vi "Set Certificate Status.vi"(8 "error in (no error)":errorcluster, 9 "Certificate Status":T1, 10 "Certificate ID":string, 11 "IoT Session in":refnum<class "IoT Session.lvclass">) -> (0 "error out":errorcluster, 3 "IoT Session out":refnum<class "IoT Session.lvclass">)   [LabVIEW 2015, in "NI_AWS_IoT.lvlib" / "IoT Session.lvclass"]
uses:
  IoT Session.lvclass
  Certificate Status.ctl
  Core/HTTP Request/Request Options.ctl
  Core/HTTP Request/Name Value Pair.ctl
  Core/HTTP Request/Region handling.ctl
  Core/HTTP Request/URL formatting.ctl
  Core/HTTP Request/HTTP Request.lvclass
  NI_AWS_IoT.lvlib
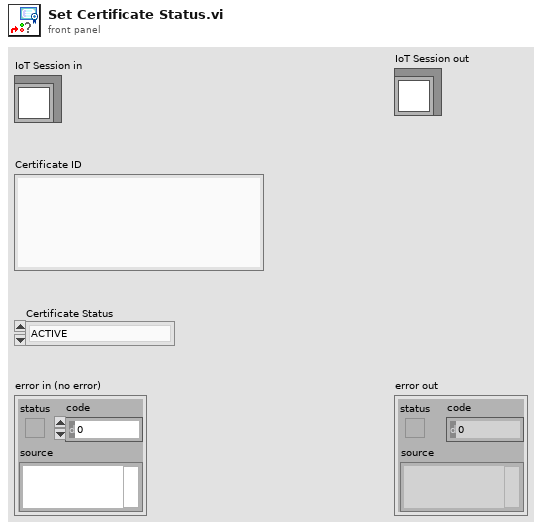
[diagram p1: front panel]
types:
  T1 = typedef "NI_AWS_IoT.lvlib/Certificate Status.ctl" = enum16{"ACTIVE", "INACTIVE", "REVOKED", "PENDING_TRANSFER", "REGISTER_INACTIVE", "PENDING_ACTIVATION"}
  T2 = typedef "NI_AWS_Core.lvlib/HTTP Request.lvclass/Name Value Pair.ctl" = cluster{"name":string, "value":string}
  T3 = typedef "NI_AWS_Core.lvlib/HTTP Request.lvclass/Request Options.ctl" = cluster{"request headers":T2[], "request parameters":T2[], "request body":string, "region handling":T4, "URL formatting":T5}
  T4 = typedef "NI_AWS_Core.lvlib/HTTP Request.lvclass/Region handling.ctl" = enum16{"use region everywhere", "use region (authentication only)", "use region (URL only)", "ignore region everwhere"}
  T5 = typedef "NI_AWS_Core.lvlib/HTTP Request.lvclass/URL formatting.ctl" = enum16{"region-", "region."}
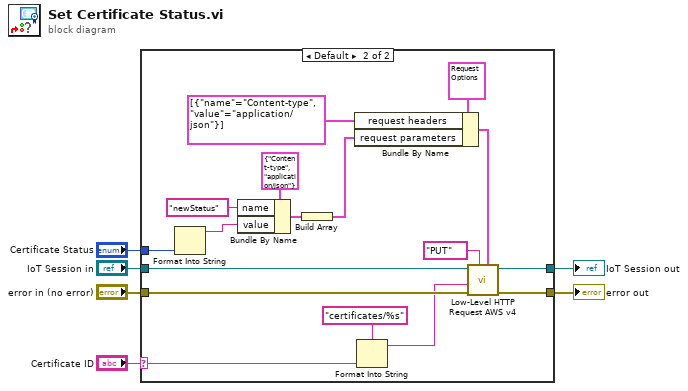
[diagram p0: block diagram]
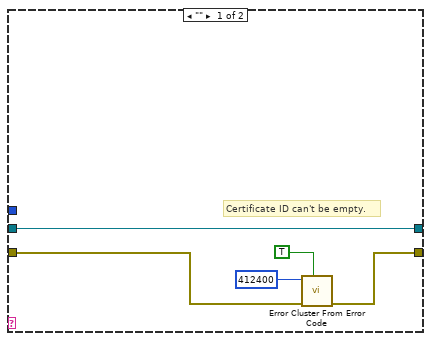
[diagram p2: hidden frame]
diagram:
  n1 = case shown="Default" "Certificate ID" {
    selector: "Certificate ID" -> [_ w19]
    tunnel: "error in (no error)" -> [w8 w28]
    tunnel: [w7 w27] -> w5
    tunnel: [w11 w26] -> w4
    tunnel: "IoT Session in" -> [w11 w25]
    tunnel: "Certificate Status" -> [_ w13]
    frame "" {
      # "Certificate ID can't be empty."
      n2 = call <vilib>:"Error Cluster From Error Code.vi"("show call chain? (False)"=TRUE, "error in (no error)"=w8, "error code (0)"=412400) -> ("error out"=w7:errorcluster)  [unwired: 6 in]
    }
    frame Default {
      n3 = Format Into String(w13) -> (resulting string=w12:string)  [unwired: 3 in, 1 out]
      n4 = Bundle By Name(cluster=T2 {"name"="Content-type", "value"="application/json"} ("Cluster"), "name"="newStatus", "value"=w12) -> (w16:T2)
      n5 = Build Array(w16) -> (w15:T2[])
      n6 = Bundle By Name(cluster=T3 {"request headers"=[], "request parameters"=[], "request body"="", "region handling"=enum."use region everywhere", "URL formatting"=enum."region."} ("Request Options"), "request headers"=T2[] [{"name"="Content-type", "value"="application/json"}], "request parameters"=w15) -> (w22:T3)
      n7 = Format Into String(format string="certificates/%s", w19) -> (resulting string=w18:string)  [unwired: 2 in, 1 out]
      n8 = call "Low-Level HTTP Request AWS v4.vi"("Request Options"=w22, "HTTP-Verb"="PUT", "error in (no error)"=w28, "URL Suffix"=w18, "AWS Core in"=w25) -> ("error out"=w27:errorcluster, "AWS Core out"=w26:refnum<class "IoT Session.lvclass">)  [unwired: 3 in, 2 out]
    }
  }
  "error out" <- w5
  "IoT Session out" <- w4
